vi "Normalize Signal Generation Parameters.vi"(0 "frequency (Hz)":dbl format="%#_6p", 1 "FPGA clock rate (Hz)":dbl=40000000.0 format="%#_6p", 5 "phase offset (deg)":dbl format="%#.6g", 7 "duty cycle (%)":dbl min=0.0 max=100.0 step=1.0, 11 "error in (no error)":errorcluster) -> (4 "frequency (periods/tick)":fxp<+,32,0> format="%.32g", 6 "phase offset (periods)":fxp<+,32,0>, 8 "duty cycle (periods)":fxp<+,32,0>, 13 "actual phase offset (deg)":dbl format="%#.6g", 14 "actual frequency (Hz)":dbl format="%#_6p", 15 "error out":errorcluster)   [LabVIEW 2020, in "NI_FpgaMspHost.lvlib"]
doc: "Converts frequency, phase, and duty cycle parameters into fixed-point units normalized to the clock rate. Use the Normalize Signal Generation Parameters VI in a host VI to convert values for the following FPGA VIs: Sine Wave Generator and Square Wave Generator."
uses:
  <vilib>/rvi/Analysis/host/Public/NI_FpgaMspHost.lvlib
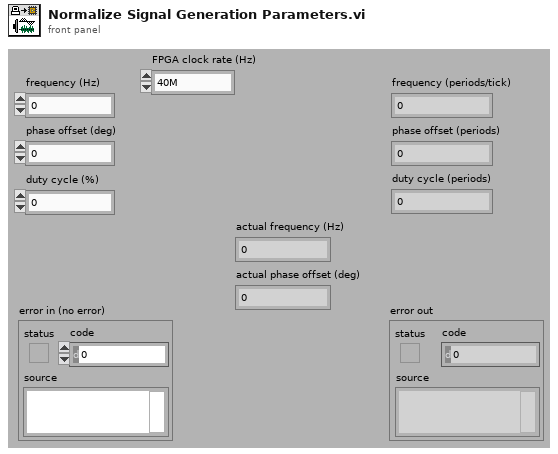
[diagram p1: front panel]
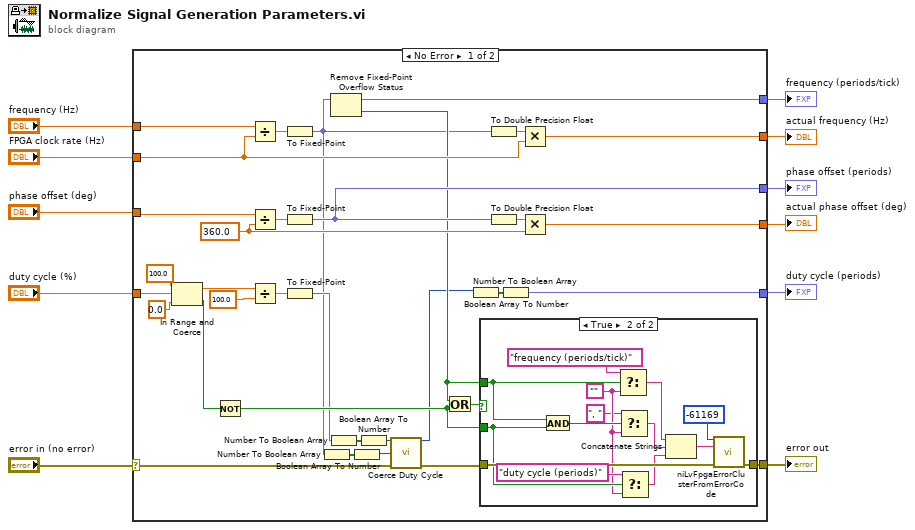
[diagram p0: block diagram]
diagram:
  n1 = case shown="No Error" "error in (no error)" {
    selector: "error in (no error)" -> [w23 w61]
    tunnel: "frequency (Hz)" -> [w45 _]
    tunnel: [w32 w61] -> w10
    tunnel: "FPGA clock rate (Hz)" -> [w43 _]
    tunnel: "phase offset (deg)" -> [w35 _]
    tunnel: "duty cycle (%)" -> [w31 _]
    tunnel: [w42 _] -> w5
    tunnel: [w41 _] -> w4
    tunnel: [w36 _] -> w3
    tunnel: [w34 _] -> w2
    tunnel: [w13 _] -> w1
    frame No Error {
      w38 = 360.0 ("y")
      n2 = In Range and Coerce(upper limit=100.0, x=w31, lower limit=0.0) -> (coerced(x)=w30:dbl, In Range?=w27:bool)
      n3 = Not(x=w27) -> (.not. x?=w24:bool)
      n4 = Divide(x=w45, y=w43) -> (x/y=w44:dbl)
      n5 = Divide(x=w35, y=w38) -> (x/y=w40:dbl)
      n6 = Divide(x=w30, y=100.0) -> (x/y=w33:dbl)
      n7 = To Fixed-Point(number=w44) -> (fixed-point=w17:fxp<+,32,0>)  [unwired: 1 out]
      n8 = To Fixed-Point(number=w40) -> (fixed-point=w34:fxp<+,32,0>)  [unwired: 1 out]
      n9 = To Fixed-Point(number=w33) -> (fixed-point=w19:fxp<+,32,0>)  [unwired: 1 out]
      n10 = Number To Boolean Array(number=w17) -> (Boolean array=w18:bool[])
      n11 = Number To Boolean Array(number=w19) -> (Boolean array=w20:bool[])
      n12 = Remove Fixed-Point Overflow Status(3:w17) -> (0:w25:bool, 1:w41:fxp<+,32,0>)
      n13 = Boolean Array To Number(Boolean array=w18) -> (number=w16:u32)
      n14 = Boolean Array To Number(Boolean array=w20) -> (number=w21:u32)
      n15 = call <vilib>:"Coerce Duty Cycle.vi"("duty cycle (scaled) in"=w21, "frequency (scaled)"=w16, "error in (no error)"=w23) -> ("duty cycle (scaled) out"=w15:u32, "error out"=w22:errorcluster)  [unwired: 11 out]
      n16 = Or(x=w25, y=w24) -> (x .or. y?=w26:bool)
      n17 = Number To Boolean Array(number=w15) -> (Boolean array=w14:bool[])
      n18 = case shown="True" w26 {
        tunnel: [w46 w60] -> w32
        tunnel: w22 -> [w46 w58]
        tunnel: w25 -> [_ w55]
        tunnel: w24 -> [_ w54]
        frame False {
        }
        frame True {
          w52 = "" ("f")
          n19 = And(x=w55, y=w54) -> (x .and. y?=w53:bool)
          n20 = Select(t="frequency (periods/tick)" ("L10N_Function Name"), s=w55, f=w52) -> (s? t:f=w50:string)
          n21 = Select(t=", ", s=w53, f=w52) -> (s? t:f=w49:string)
          n22 = Select(t="duty cycle (periods)" ("L10N_Function Name"), s=w54, f=w52) -> (s? t:f=w48:string)
          n23 = Concatenate Strings(w50, w49, w48) -> (w47:string)
          n24 = call <vilib>:"niLvFpgaErrorClusterFromErrorCode.vi"("error code"=-61169, "function name"=w47, "error in"=w58) -> ("error out"=w60:errorcluster)  [unwired: 4 in, 8 out]
        }
      }
      n25 = To Double Precision Float(number=w17) -> (double precision float=w39:dbl)
      n26 = To Double Precision Float(number=w34) -> (double precision float=w37:dbl)
      n27 = Boolean Array To Number(Boolean array=w14) -> (number=w13:fxp<+,32,0>)
      n28 = Multiply(x=w39, y=w43) -> (x*y=w42:dbl)
      n29 = Multiply(x=w37, y=w38) -> (x*y=w36:dbl)
    }
    frame Error {
    }
  }
  "frequency (periods/tick)" <- w4
  "error out" <- w10
  "duty cycle (periods)" <- w1
  "phase offset (periods)" <- w2
  "actual frequency (Hz)" <- w5
  "actual phase offset (deg)" <- w3
